vi "system stop.vi"() -> ()   [LabVIEW 2021]
panel:
  out "KB":u8[](array[numeric])
  out "KA":u8[](array[numeric])
  in  "Do Nothing":bool
  out "USRP2 EnvRSSI in dBm":dbl
  out "USRP1 EnvRSSI in dBm":dbl
  out "USRP2 Phase deg":dbl
  out "USRP1 Phase deg":dbl
  out "USRP2 Freq Offset in Hz":dbl
  out "USRP1 Freq Offset in Hz":dbl
  out "USRP2 volt in V":dbl
  out "USRP1 volt in V":dbl
  out "USRP2 RSSI saved":bool
  out "USRP1 RSSI saved":bool
  in  "Change Freq":bool
  out "System Stop":bool
  in  "USRP2 stop":bool
  in  "CarrierFrequency":dbl=2400000000.0
  out "USRP2 Rx Complete":bool
  out "USRP1 Rx Complete":bool
  out "USRP2 Tx Complete":bool
  out "USRP1 Tx Complete":bool
  in  "USRP2 Tx":bool
  in  "USRP1 Tx":bool
  in  "USRP2 Pkt Rx":bool
  in  "USRP1 Tx Stop":bool
  in  "stop":bool
  in  "USRP2 Tx Stop":bool
  out "Transmitted Flag":bool
  in  "system stop Spectrum Analyzer":bool
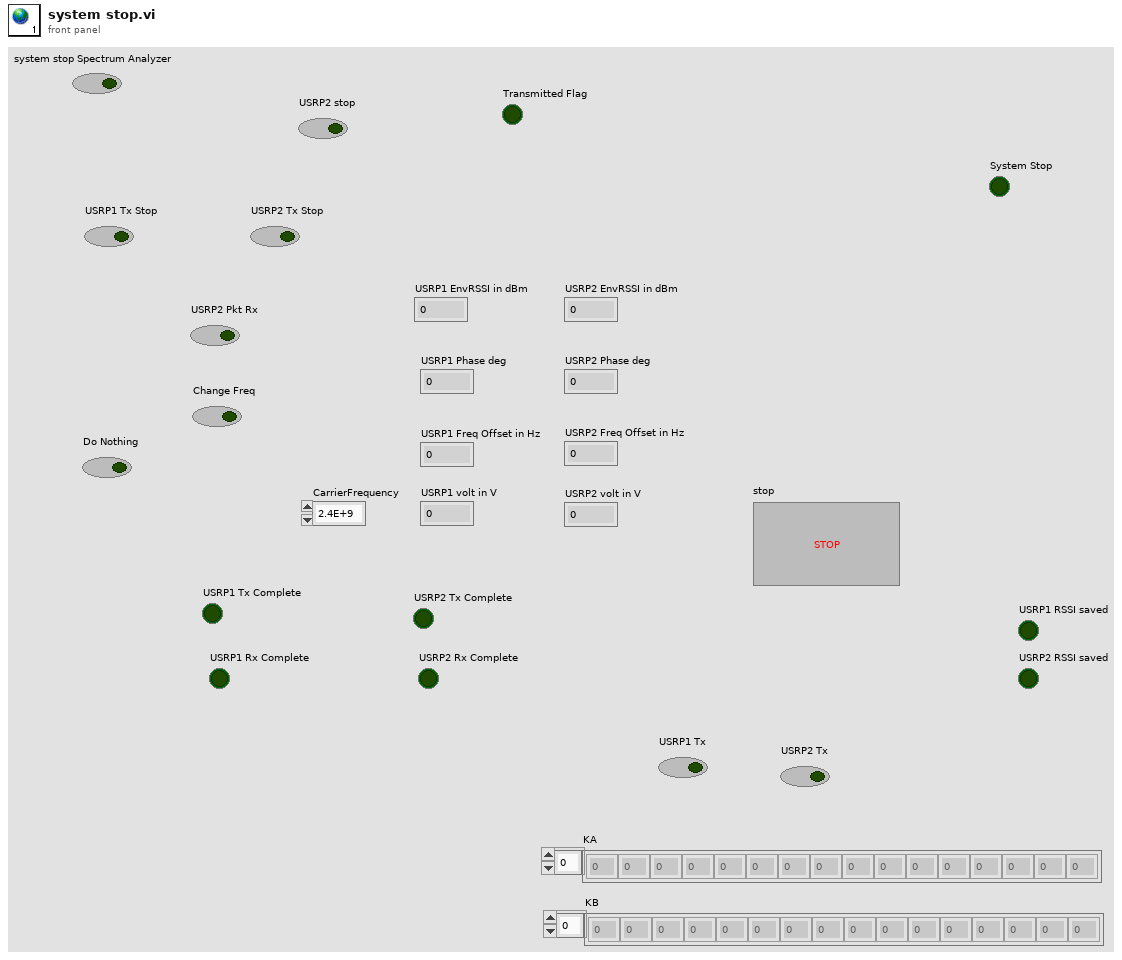
[diagram p1: front panel]
diagram:
